vi "Teleop.vi"(10 "Match Info":T1={"Autonomous Elapsed Seconds"=0.0, "TeleOp Elapsed Seconds"=0.0, "Disabled Elapsed Seconds"=0.0, "Visited Autonomous"=FALSE, "Visited TeleOp"=FALSE, "Visited Disabled"=FALSE, "Autonomous Settings"={"Autonomous Style"=enum."Independent", "VI Refnum"=refnum}}, 11 "Call Context":T2) -> ()   [LabVIEW 2019]
doc: "This VI is called for each TeleOp packet received from the DS where the robot is not disabled. It is often used to read from the joysticks and update I/O or to update setpoints for timed control loops. It should complete and return within 20 milliseconds or it may miss DS packets."
uses:
  <vilib>/Rock Robotics/WPI/DriverStation/WPI_DriverStationDerivedRobotMode.ctl
  <vilib>/Rock Robotics/WPI/DriverStation/WPI_DriverStationMatch Info.ctl
  <vilib>/Rock Robotics/WPI/Utilities/WPI_GetSetVariantRefNum.vi
  Robot Global Data.vi
  <vilib>/Rock Robotics/Network Tables/NT Write Number.vi
  <vilib>/Rock Robotics/Network Tables/NT Write Numeric Array.vi
  <vilib>/Rock Robotics/Network Tables/NT Write Boolean Array.vi
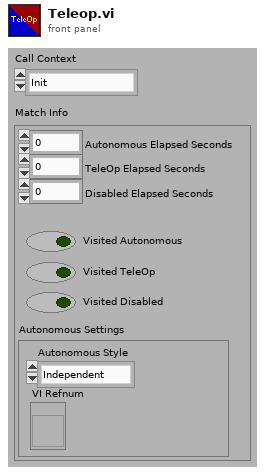
[diagram p1: front panel]
types:
  T1 = typedef "WPI_DriverStationMatch Info.ctl" = cluster{"Autonomous Elapsed Seconds":dbl, "TeleOp Elapsed Seconds":dbl, "Disabled Elapsed Seconds":dbl, "Visited Autonomous":bool, "Visited TeleOp":bool, "Visited Disabled":bool, "Autonomous Settings":cluster{"Autonomous Style":enum16{"Iterative", "Independent"}, "VI Refnum":refnum<vi>}}
  T2 = typedef "WPI_DriverStationDerivedRobotMode.ctl" = enum16{"Init", "Execute", "Stop"}
  T3 = typedef "WPI_JoystickDevRef.ctl" = cluster{"Device":T4}
  T4 = typedef "WPI_JoystickDeviceEnum.ctl" = enum16{"USB 0", "USB 1", "USB 2", "USB 3", "USB 4", "USB 5"}
  T5 = typedef "WPI_RobotDriveDevRef.ctl" = cluster{"DevStatus":errorcluster, "Motors[]":T6[], "Square Inputs":bool, "Max Output":dbl}
  T6 = typedef "WPI_MotorControlDeviceRef.ctl" = cluster{"DeviceStatus":errorcluster, "Type":T7, "PWM":cluster{"PWM Channel":T8, "DeadBand":T9}, "CAN":cluster{"Device Number":u8, "SetOutput VI Ref":variant, "GetOutput VI Ref":variant, "Enable VI Ref":variant, "Disable VI Ref":variant, "Data":variant}, "Invert":bool, "DIO PWM":cluster{"PWM \"Enable\" Channel":T8, "DIOChannel":T10, "PWM Rate":dbl}}
  T7 = typedef "WPI_MotorControlType.ctl" = enum16{"PWM", "CAN", "DIO PWM"}
  T8 = typedef "FPGA_DIOPWMChannel.ctl" = enum8{"PWM 0", "PWM 1", "PWM 2", "PWM 3", "PWM 4", "PWM 5", "PWM 6", "PWM 7", "PWM 8", "PWM 9", "PWM MXP 0", "PWM MXP 1", "PWM MXP 2", "PWM MXP 3", "PWM MXP 4", "PWM MXP 5", "PWM MXP 6", "PWM MXP 7", "PWM MXP 8", "PWM MXP 9", "Invalid"}
  T9 = typedef "WPI_PWMDeadband.ctl" = cluster{"Name":string, "maxPositivePwm":i32, "minPositivePwm":i32, "centerPwm":i32, "maxNegativePwm":i32, "minNegativePwm":i32, "angularRange":u16}
  T10 = typedef "FPGA_DIOChannel.ctl" = enum8{"DIO 0", "DIO 1", "DIO 2", "DIO 3", "DIO 4", "DIO 5", "DIO 6", "DIO 7", "DIO 8", "DIO 9", "DIO MXP 0", "DIO MXP 1", "DIO MXP 2", "DIO MXP 3", "DIO MXP 4", "DIO MXP 5", "DIO MXP 6", "DIO MXP 7", "DIO MXP 8", "DIO MXP 9", "DIO MXP 10", "DIO MXP 11", "DIO MXP 12", "DIO MXP 13", "DIO MXP 14", "DIO MXP 15", "SPI Port CS1", "SPI Port CS2", "SPI Port CS3", "SPI Port MISO", "SPI Port MOSI", "Invalid"}
  T11 = cluster{"JoystickDevRef":T3, "RobotDriveDevRef":T5}
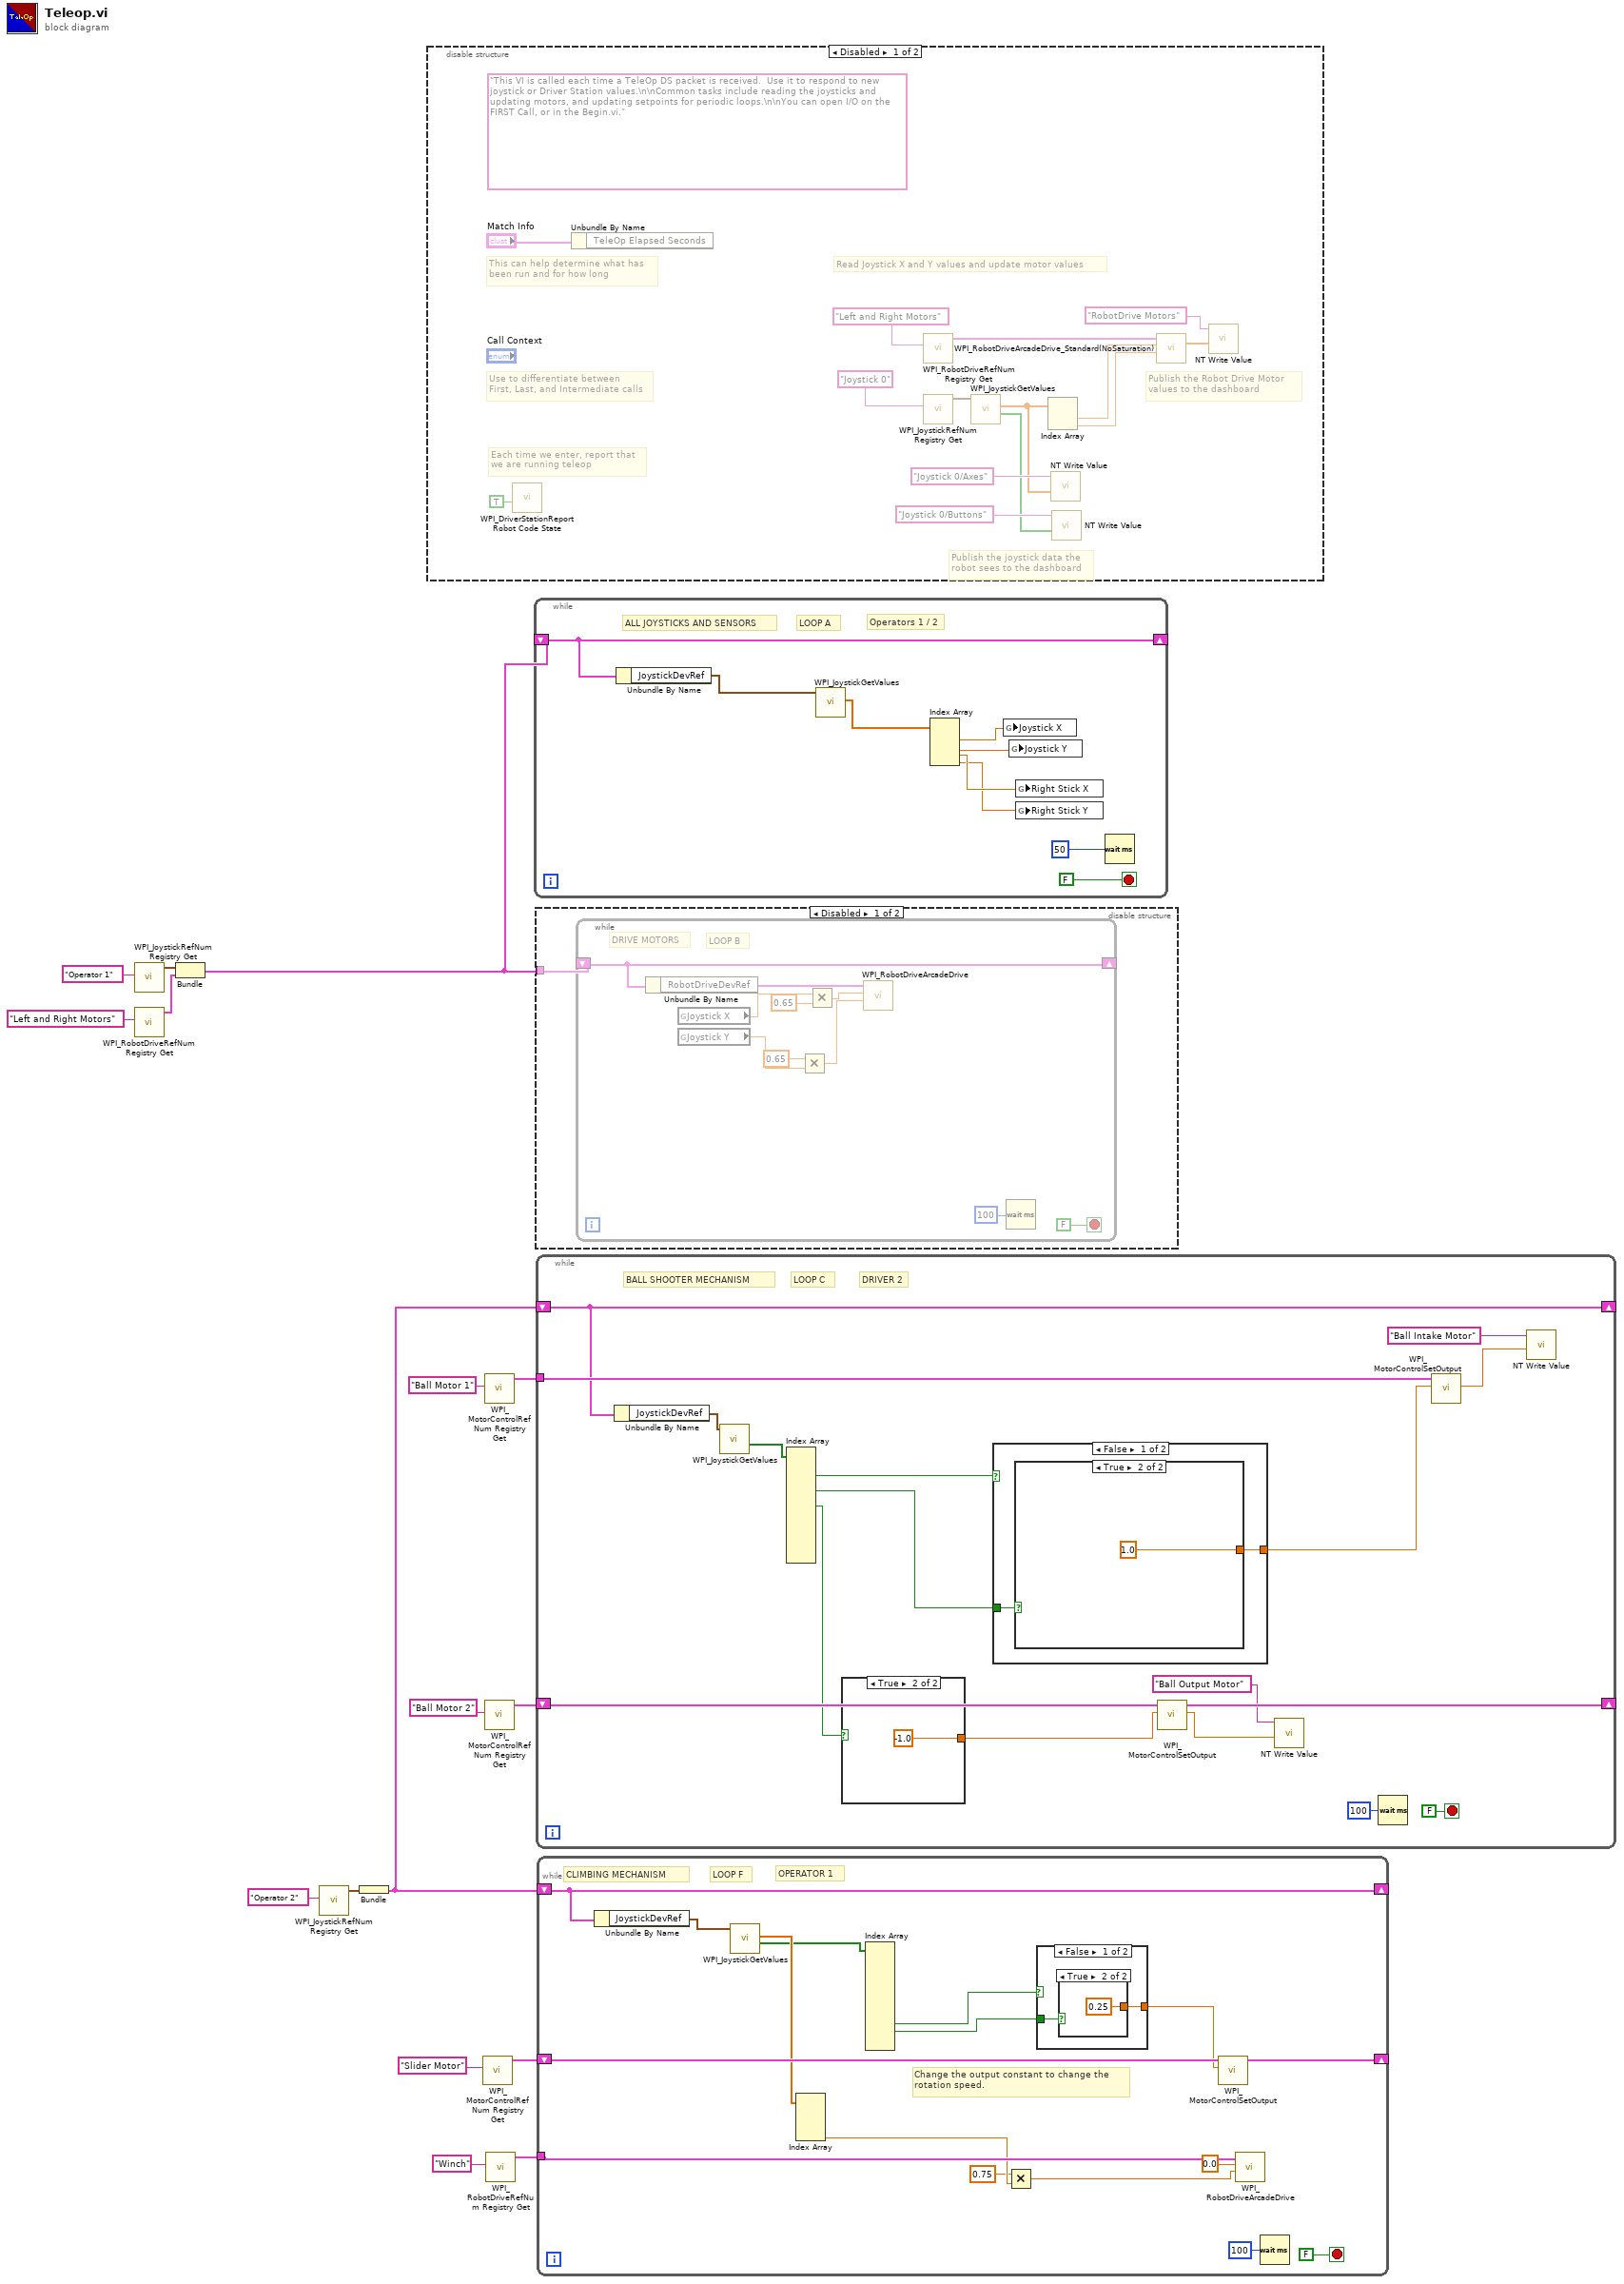
[diagram p0: block diagram]
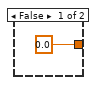
[diagram p2: hidden frame]
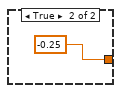
[diagram p3: hidden frame]
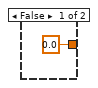
[diagram p6: hidden frame]
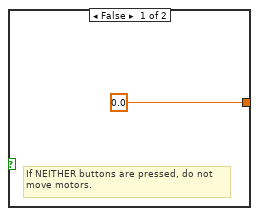
[diagram p7: hidden frame]
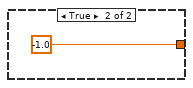
[diagram p8: hidden frame]
diagram:
  n1 = call <vilib>:"WPI_JoystickRefNum Registry Get.vi"("refnum name"="Operator 1") -> ("JoystickDevRef"=w14:T3)  [unwired: 1 in, 9 out]
  n2 = call <vilib>:"WPI_RobotDriveRefNum Registry Get.vi"("refnum name"="Left and Right Motors") -> ("RobotDriveDevRef"=w13:T5)  [unwired: 1 in, 9 out]
  n3 = Bundle("JoystickDevRef"=w14, "RobotDriveDevRef"=w13) -> (w3:T11)  [unwired: 1 out]
  n4 = call <vilib>:"WPI_JoystickRefNum Registry Get.vi"("refnum name"="Operator 2") -> ("JoystickDevRef"=w5:T3)  [unwired: 9 in, 1 out]
  n5 = Bundle("JoystickDevRef"=w5) -> (w2:cluster{"JoystickDevRef":T3})  [unwired: 1 in]
  n6 = disable-structure shown="Disabled" {
    frame Disabled {
      (unwired) "This VI is called each time a TeleOp DS packet is received.  Use it to respond to new joystick or Driver Station values.\n\nCommon tasks include reading the joysticks and updating motors, and updating setpoints for periodic loops.\n\nYou can open I/O on the FIRST Call, or in the Begin.vi."
      # "Publish the Robot Drive Motor\nvalues to the dashboard"
      # "Publish the joystick data the\nrobot sees to the dashboard"
      # "Each time we enter, report that\nwe are running teleop"
      # "Use to differentiate between\nFirst, Last, and Intermediate calls"
      # "This can help determine what has\nbeen run and for how long"
      # "Read Joystick X and Y values and update motor values"
      n7 = call <vilib>:"WPI_DriverStationReport Robot Code State.vi"("TeleOp"=TRUE ("Autonomous")) -> ()  [unwired: 10 in, 1 out]
      n8 = Unbundle By Name("Match Info") -> ()  [unwired: 1 out]
      n9 = call <vilib>:"WPI_RobotDriveRefNum Registry Get.vi"("refnum name"="Left and Right Motors") -> ("RobotDriveDevRef"=w28:T5)  [unwired: 1 in, 9 out]
      n10 = call <vilib>:"WPI_JoystickRefNum Registry Get.vi"("refnum name"="Joystick 0") -> ("JoystickDevRef"=w25:T3)  [unwired: 1 in, 9 out]
      n11 = call <vilib>:"WPI_JoystickGetValues.vi"("JoystickDevRef"=w25) -> ("Buttons"=w19:bool[], "Axes"=w20:dbl[])  [unwired: 6 in, 3 out]
      n12 = Index Array(array=w20) -> (element #1=w27:dbl, element #2=w23:dbl)  [unwired: 2 in]
      n13 = call-poly <vilib>:"NT Write Value.vi"("Numeric Array"=w20, "Name"="Joystick 0/Axes") -> ()  [unwired: 9 in, 1 out]
      n14 = call-poly <vilib>:"NT Write Value.vi"("Boolean Array"=w19, "Name"="Joystick 0/Buttons") -> ()  [unwired: 9 in, 1 out]
      n15 = call <vilib>:"WPI_RobotDriveArcadeDrive_Standard(NoSaturation).vi"("Y axis value"=w23, "X axis value"=w27, "RobotDriveDevRef"=w28) -> ("Motor Values"=w18:dbl[])  [unwired: 1 in, 7 out]
      n16 = call-poly <vilib>:"NT Write Value.vi"("Numeric Array"=w18, "Name"="RobotDrive Motors") -> ()  [unwired: 9 in, 1 out]
    }
    frame Enabled {
    }
  }
  n17 = call <vilib>:"WPI_MotorControlRefNum Registry Get.vi"("refnum name"="Slider Motor") -> ("MotorControlDevRef"=w8:T6)  [unwired: 9 in, 1 out]
  n18 = call <vilib>:"WPI_MotorControlRefNum Registry Get.vi"("refnum name"="Ball Motor 1") -> ("MotorControlDevRef"=w11:T6)  [unwired: 9 in, 1 out]
  n19 = call <vilib>:"WPI_MotorControlRefNum Registry Get.vi"("refnum name"="Ball Motor 2") -> ("MotorControlDevRef"=w9:T6)  [unwired: 9 in, 1 out]
  n20 = call <vilib>:"WPI_RobotDriveRefNum Registry Get.vi"("refnum name"="Winch") -> ("RobotDriveDevRef"=w4:T5)  [unwired: 9 in, 1 out]
  n21 = while {
    shift-right: [w38] -> _
    shift-left: w3 -> [w38]
    stop <- FALSE stop-if-true
    # "Operators 1 / 2"
    # "LOOP A"
    # "ALL JOYSTICKS AND SENSORS"
    n22 = Unbundle By Name(w38) -> ("JoystickDevRef"=w37:T3)
    n23 = call <vilib>:"WPI_JoystickGetValues.vi"("JoystickDevRef"=w37) -> ("Axes"=w36:dbl[])  [unwired: 6 in, 4 out]
    n24 = Index Array(array=w36) -> (element #1=w34:dbl, element #2=w35:dbl, element #3=w32:dbl, element #4=w31:dbl)  [unwired: 4 in]
    n25 = global write "Robot Global Data.vi" "Joystick X"(w34) -> ()
    n26 = global write "Robot Global Data.vi" "Joystick Y"(w35) -> ()
    n27 = global write "Robot Global Data.vi" "Right Stick X"(w32) -> ()
    n28 = global write "Robot Global Data.vi" "Right Stick Y"(w31) -> ()
    n29 = Wait (ms)(milliseconds to wait=u32 50) -> ()  [unwired: 1 out]
  }
  n30 = disable-structure shown="Disabled" {
    disable-tunnel: w3 -> [w40 _]
    frame Disabled {
      n31 = while {
        shift-right: [w48] -> _
        shift-left: w40 -> [w48]
        stop <- FALSE stop-if-true
        # "DRIVE MOTORS"
        # "LOOP B"
        n32 = Unbundle By Name(w48) -> ("RobotDriveDevRef"=w47:T5)
        n33 = global read "Robot Global Data.vi" "Joystick X"() -> (w45:dbl)
        n34 = global read "Robot Global Data.vi" "Joystick Y"() -> (w46:dbl)
        n35 = Multiply(x=0.65, y=w46) -> (x*y=w42:dbl)
        n36 = Multiply(x=w45, y=0.65) -> (x*y=w41:dbl)
        n37 = call-poly <vilib>:"WPI_RobotDriveArcadeDrive.vi"("Y axis value"=w42, "X axis value"=w41, "RobotDriveDevRef"=w47) -> ()  [unwired: 6 in, 3 out]
        n38 = Wait (ms)(milliseconds to wait=u32 100) -> ()  [unwired: 1 out]
      }
    }
    frame Enabled {
    }
  }
  n39 = while {
    tunnel: w11 -> [w65]
    shift-right: [w61] -> _
    shift-left: w9 -> [w62]
    shift-right: [w54] -> _
    shift-left: w2 -> [w54]
    stop <- FALSE stop-if-true
    # "DRIVER 2"
    # "LOOP C"
    # "BALL SHOOTER MECHANISM"
    n40 = Unbundle By Name(w54) -> ("JoystickDevRef"=w53:T3)
    n41 = call <vilib>:"WPI_JoystickGetValues.vi"("JoystickDevRef"=w53) -> ("Buttons"=w63:bool[])  [unwired: 6 in, 4 out]
    n42 = Index Array(array=w63) -> (element #2=w52:bool, element #4=w51:bool, element #6=w59:bool)  [unwired: 13 in, 10 out]
    n43 = case shown="True" w59 {
      tunnel: [0.0 ("Output") -1.0 ("Output")] -> w60
      frame False {
      }
      frame True {
      }
    }
    n44 = case shown="False" w52 {
      tunnel: [w71 -1.0 ("Output")] -> w64
      tunnel: w51 -> [w70 _]
      frame False {
        n45 = case shown="True" w70 {
          tunnel: [0.0 ("Output") 1.0 ("Output")] -> w71
          frame False {
            # "If NEITHER buttons are pressed, do not\nmove motors."
          }
          frame True {
          }
        }
      }
      frame True {
      }
    }
    n46 = call <vilib>:"WPI_MotorControlSetOutput.vi"("Output"=w60, "MotorControlDevRef"=w62) -> ("Motor Output"=w56:dbl, "MotorControlDevRef"=w61:T6)  [unwired: 7 in, 1 out]
    n47 = call-poly <vilib>:"NT Write Value.vi"("Numeric"=w56, "Name"="Ball Output Motor") -> ()  [unwired: 9 in, 1 out]
    n48 = Wait (ms)(milliseconds to wait=u32 100) -> ()  [unwired: 1 out]
    n49 = call <vilib>:"WPI_MotorControlSetOutput.vi"("Output"=w64, "MotorControlDevRef"=w65) -> ("Motor Output"=w58:dbl)  [unwired: 7 in, 2 out]
    n50 = call-poly <vilib>:"NT Write Value.vi"("Numeric"=w58, "Name"="Ball Intake Motor") -> ()  [unwired: 9 in, 1 out]
  }
  n51 = while {
    shift-right: [w78] -> _
    shift-left: w8 -> [w90]
    tunnel: w4 -> [w85]
    shift-right: [w80] -> _
    shift-left: w2 -> [w80]
    stop <- FALSE stop-if-true
    # "Change the output constant to change the\nrotation speed."
    # "OPERATOR 1"
    # "LOOP F"
    # "CLIMBING MECHANISM"
    n52 = Unbundle By Name(w80) -> ("JoystickDevRef"=w79:T3)
    n53 = call <vilib>:"WPI_JoystickGetValues.vi"("JoystickDevRef"=w79) -> ("Buttons"=w83:bool[], "Axes"=w86:dbl[])  [unwired: 6 in, 3 out]
    n54 = Index Array(array=w86) -> (element #4=w84:dbl)  [unwired: 4 in, 3 out]
    n55 = Index Array(array=w83) -> (element #9=w82:bool, element #10=w81:bool)  [unwired: 12 in, 10 out]
    n56 = Multiply(x=0.75, y=w84) -> (x*y=w76:dbl)
    n57 = case shown="False" w82 {
      tunnel: [w92 -0.25 ("Output")] -> w88
      tunnel: w81 -> [w91 _]
      frame False {
        n58 = case shown="True" w91 {
          tunnel: [0.0 ("Output") 0.25 ("Output")] -> w92
          frame False {
          }
          frame True {
          }
        }
      }
      frame True {
      }
    }
    n59 = call <vilib>:"WPI_MotorControlSetOutput.vi"("Output"=w88, "MotorControlDevRef"=w90) -> ("MotorControlDevRef"=w78:T6)  [unwired: 7 in, 2 out]
    n60 = call-poly <vilib>:"WPI_RobotDriveArcadeDrive.vi"("Y axis value"=w76, "X axis value"=0.0, "RobotDriveDevRef"=w85) -> ()  [unwired: 6 in, 3 out]
    n61 = Wait (ms)(milliseconds to wait=u32 100) -> ()  [unwired: 1 out]
  }
